vi "Counter Driver.vi"(8 "error in":errorcluster, 9 "Characters to Write":string="*IDN?", 10 "Operation":T1(ring), 11 "GPIB Address":u32=3) -> (0 "Error Out":errorcluster, 1 "Characters Read":string, 3 "GPIB Address Out":i32)   [LabVIEW 2009]
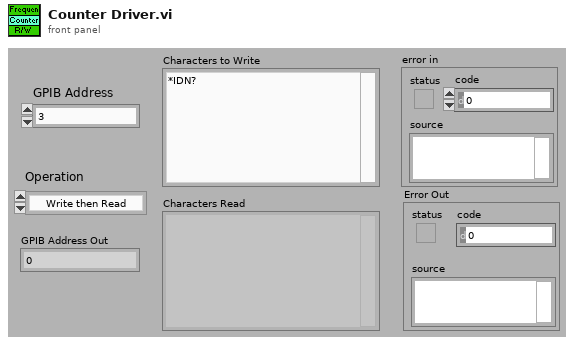
[diagram p1: front panel]
types:
  T1 = enum16{"Write then Read", "Write to Instr", "Read from Instr"}
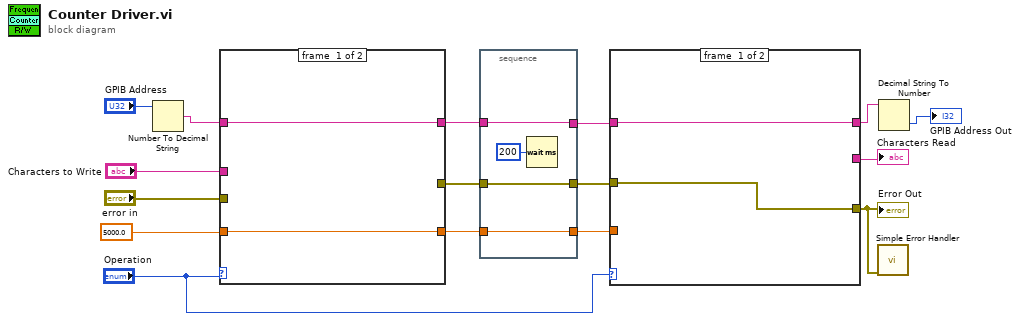
[diagram p0: block diagram]
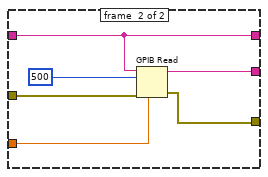
[diagram p2: hidden frame]
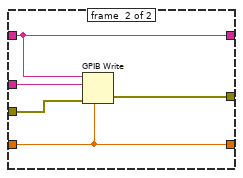
[diagram p3: hidden frame]
diagram:
  n1 = Number To Decimal String(number="GPIB Address") -> (decimal integer string=w4:string)  [unwired: 1 out]
  n2 = case shown="\"Write then Read\", \"Write to Instr\"" "Operation" {
    tunnel: w4 -> [w18 w22]
    tunnel: "Characters to Write" -> [_ w23]
    tunnel: 5000.0 ("Timeout (ms)") -> [w17 w21]
    tunnel: [w18 w22] -> w15
    tunnel: [w17 w21] -> w11
    tunnel: [_ w20] -> w13
    tunnel: "error in" -> [_ w19]
    frame #0 {
    }
    frame #1 {
      n3 = GPIB Write(0:w22, 1:w23, 3:w19, 4:w21) -> (6:w20:errorcluster)  [unwired: 1 in, 1 out]
    }
  }
  n4 = stacked-sequence {
    tunnel: w15 -> [w27]
    tunnel: [w27] -> w14
    tunnel: w13 -> [w26]
    tunnel: [w26] -> w12
    tunnel: w11 -> [w25]
    tunnel: [w25] -> w10
    frame #0 {
      n5 = Wait (ms)(milliseconds to wait=u32 200) -> ()  [unwired: 1 out]
    }
  }
  n6 = case shown="\"Write then Read\", \"Read from Instr\"" "Operation" {
    tunnel: w14 -> [w28 w30]
    tunnel: [_ w35] -> w1
    tunnel: w10 -> [_ w34]
    tunnel: w12 -> [w29 w33]
    tunnel: [w29 w32] -> w9
    tunnel: [w28 w30] -> w3
    frame #0 {
    }
    frame #1 {
      n7 = GPIB Read(0:w30, 1:500 ("# Bytes to Read"), 3:w33, 4:w34) -> (5:w35:string, 7:w32:errorcluster)  [unwired: 1 in, 1 out]
    }
  }
  "Characters Read" <- w1
  "Error Out" <- w9
  n8 = call <vilib>:"Simple Error Handler.vi"("error in (no error)"=w9) -> ()  [unwired: 1 in, 8 out]
  n9 = Decimal String To Number(string=w3) -> (number=→"GPIB Address Out":i32)  [unwired: 3 out]
